vi "turret.vi"(1 "rate in (-1 to 1)":dbl) -> (0 "Output":dbl)   [LabVIEW 2011]
doc: "Closed loop turret control. Loop is closed on rate, make sure that the turret turn smoothly. This VI also containts some safeties that prevent the turret from rotating too far, and catches a loss of encoder signal and then stops the movement. Implemented after (expensive) lessons learned last year.s"
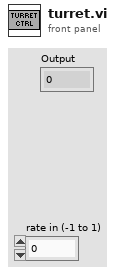
[diagram p1: front panel]
types:
  T1 = typedef "WPI_EncoderDevRef.ctl" = cluster{"DevStatus":errorcluster, "EncoderIndex":T2, "CounterIndex":T3, "DistancePerCount":dbl, "Decoding Type":T4}
  T2 = typedef "FPGA_EncoderIdx.ctl" = enum8{"Enc 0", "Enc 1", "Enc 2", "Enc 3", "Invalid"}
  T3 = typedef "FPGA_CounterCtrSystemIndex.ctl" = enum8{"Ctr 0", "Ctr 1", "Ctr 2", "Ctr 3", "Ctr 4", "Ctr 5", "Ctr 6", "Ctr 7", "Invalid"}
  T4 = typedef "WPI_EncoderType.ctl" = enum16{"1x", "2x", "4x"}
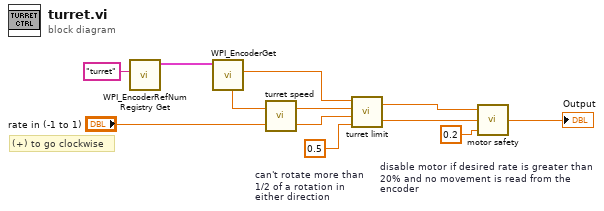
[diagram p0: block diagram]
diagram:
  w1 = 0.2  # disable motor if desired rate is greater than 20% and no movement is read from the encoder
  w4 = 0.5  # can't rotate more than 1/2 of a rotation in either direction
  # "(+) to go clockwise"
  n1 = call <vilib>:"WPI_EncoderRefNum Registry Get.vi"("refnum name"="turret") -> ("EncoderDevRef"=w11:T1)  [unwired: 9 in, 1 out]
  n2 = call <vilib>:"WPI_EncoderGet.vi"("EncoderDevRef"=w11) -> ("Distance"=w7:dbl, "Rate"=w8:dbl)  [unwired: 5 in, 4 out]
  n3 = call "turret speed.vi"("rate in (-1 to 1)"="rate in (-1 to 1)", "Current Rate"=w8) -> ("output speed"=w5:dbl, "current filtered rate"=w6:dbl)
  n4 = call "turret limit.vi"("limit"=w4, "output speed"=w5, "Current Rate in"=w6, "Distance"=w7) -> ("limited output speed"=w2:dbl, "Current Rate out"=w3:dbl)
  n5 = call "motor safety.vi"("no signal cutoff rate"=w1, "Motor Output"=w2, "Current Rate"=w3) -> ("Safe Motor Output"=→"Output":dbl)
